vi "Check and Run.vi"(11 "Error In":errorcluster) -> (15 "Error":errorcluster)   [LabVIEW 2020]
uses:
  <vilib>/vision/Image Controls.llb/IMAQ Image.ctl
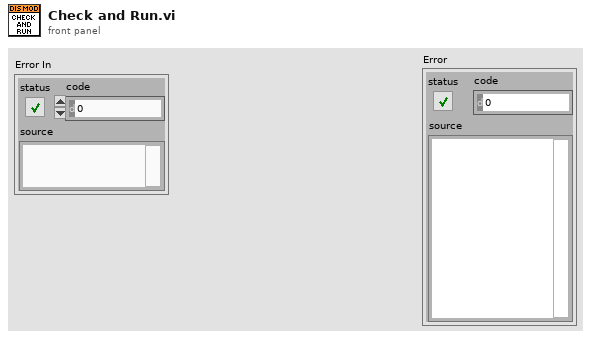
[diagram p1: front panel]
types:
  T1 = typedef "IMAQ Image.ctl" = refnum<image>
  T2 = enum32{"Bad", "Idle", "Run top level", "Running"}
  T3 = enum32{"Invalid", "Standard", "Closed", "Hidden", "Minimized", "Maximized"}
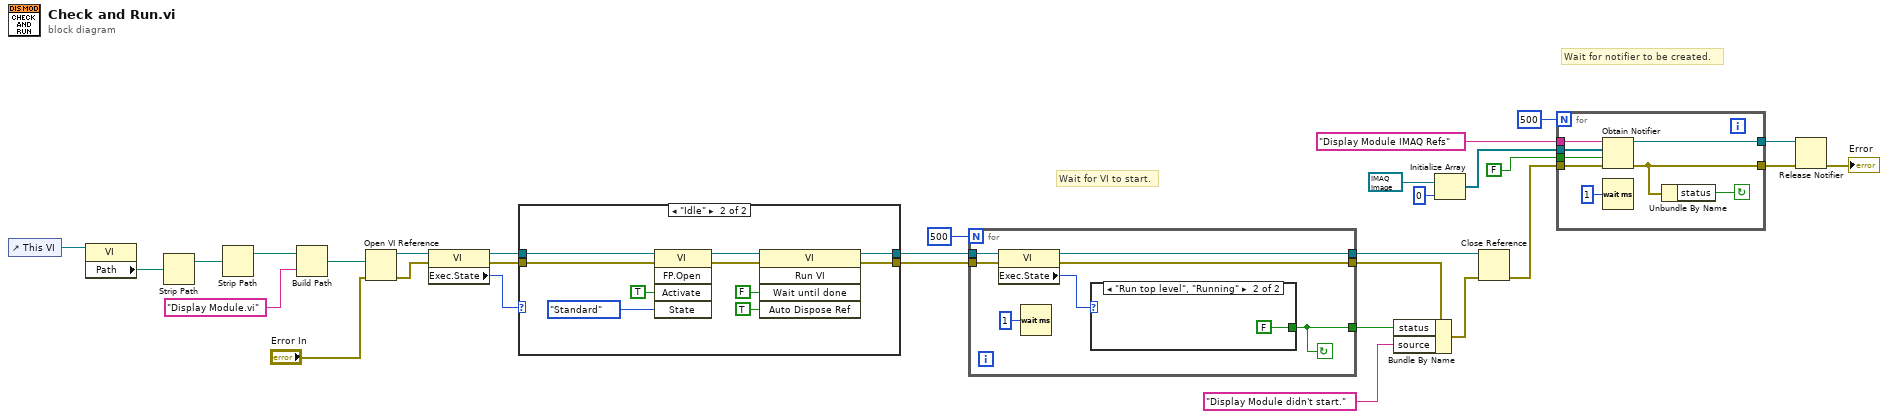
[diagram p0: block diagram]
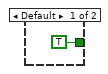
[diagram p2: hidden frame]
diagram:
  # "Wait for notifier to be created."
  # "Wait for VI to start."
  n1 = control-ref of="This VI"() -> (w30:refnum<vi>)
  n2 = property class="VI"(reference=w30) -> ("Path"=w29:path)  [unwired: 1 in, 2 out]
  n3 = Strip Path(path=w29) -> (stripped path=w28:path)  [unwired: 1 out]
  n4 = Strip Path(path=w28) -> (stripped path=w27:path)  [unwired: 1 out]
  n5 = Build Path(base path=w27, name or relative path="Display Module.vi") -> (appended path=w23:path)
  n6 = Open VI Reference(vi path=w23, error in (no error)="Error In") -> (vi reference=w25:refnum<vi>, error out=w22:errorcluster)  [unwired: 4 in]
  n7 = property class="VI"(reference=w25, error in=w22) -> (reference out=w21:refnum<vi>, error out=w20:errorcluster, "Exec.State"=w24:T2)
  n8 = case shown="\"Idle\"" w24 {
    tunnel: w20 -> [w32 w36]
    tunnel: [w32 w34] -> w17
    tunnel: w21 -> [w31 w37]
    tunnel: [w31 w33] -> w18
    frame Default {
    }
    frame "Idle" {
      n9 = invoke class="VI" method="FP.Open"(reference=w37, error in=w36, "Activate"=TRUE ("Activate?"), "State"=T3."Standard") -> (reference out=w40:refnum<vi>, error out=w35:errorcluster)  [unwired: 1 in, 3 out]
      n10 = invoke class="VI" method="Run VI"(reference=w40, error in=w35, "Wait until done"=FALSE ("Wait Until Done"), "Auto Dispose Ref"=TRUE ("Auto Dispose Reference")) -> (reference out=w33:refnum<vi>, error out=w34:errorcluster)  [unwired: 1 in, 3 out]
    }
  }
  n11 = for {
    N: 500 -> [_]
    tunnel: w18 -> [w48]
    tunnel: w17 -> [w47]
    tunnel: [w45] -> w16
    tunnel: [w44] -> w15
    tunnel: [w43] -> w13
    stop <- w43 continue-if-true
    n12 = property class="VI"(reference=w48, error in=w47) -> (reference out=w45:refnum<vi>, error out=w44:errorcluster, "Exec.State"=w46:T2)
    n13 = Wait (ms)(milliseconds to wait=u32 1) -> ()  [unwired: 1 out]
    n14 = case shown="\"Run top level\", \"Running\"" w46 {
      tunnel: [TRUE FALSE] -> w43
      frame Default {
      }
      frame "Run top level", "Running" {
      }
    }
  }
  n15 = Bundle By Name(cluster=w15, "status"=w13, "source"="Display Module didn't start.") -> (w14:errorcluster)
  n16 = Initialize Array(T1 refnum ("New Image"), 0 ("dimension size")) -> (w6:T1[])
  n17 = Close Reference(reference=w16, error in (no error)=w14) -> (error out=w5:errorcluster)
  n18 = for {
    N: 500 -> [_]
    tunnel: "Display Module IMAQ Refs" ("name (unnamed)") -> [w59]
    tunnel: FALSE ("create if not found? (T)") -> [w58]
    tunnel: w6 -> [w57]
    tunnel: w5 -> [w56]
    tunnel: [w53] -> w2
    tunnel: [w52] -> w3
    stop <- w54 continue-if-true
    n19 = Obtain Notifier(name (unnamed)=w59, notification data type=w57, create if not found? (T)=w58, error in (no error)=w56) -> (notifier out=w52:refnum<notifier>, error out=w53:errorcluster)  [unwired: 1 out]
    n20 = Wait (ms)(milliseconds to wait=u32 1) -> ()  [unwired: 1 out]
    n21 = Unbundle By Name(w53) -> ("status"=w54:bool)
  }
  n22 = Release Notifier(notifier=w3, error in (no error)=w2) -> (error out=→"Error":errorcluster)  [unwired: 1 in, 2 out]
